vi "stop_gb_test_if_hp_test_fail.vi"(8 "error in (no error)":errorcluster, 9 "Message Queues in":T1, 11 "Pass/Fail":cluster{"PASS":bool, "FAIL":bool}) -> (0 "error out":errorcluster, 1 "Message Queues out":T1, 3 "Fail?":bool)   [LabVIEW 2015]
uses:
  support/Message Queue/All Message Queues.ctl
  support/Message Queue/Message Cluster.ctl
  support/Message Queue/Enqueue Message (Array).vi
  support/Message Queue/Message Queue.lvlib
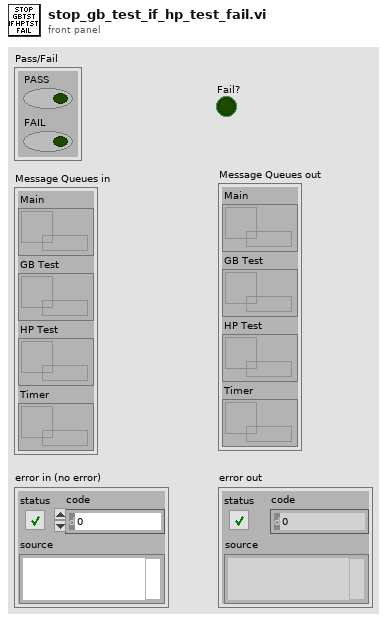
[diagram p1: front panel]
types:
  T1 = typedef "Message Queue.lvlib/All Message Queues.ctl" = cluster{"Main":refnum<queue>, "GB Test":refnum<queue>, "HP Test":refnum<queue>, "Timer":refnum<queue>}
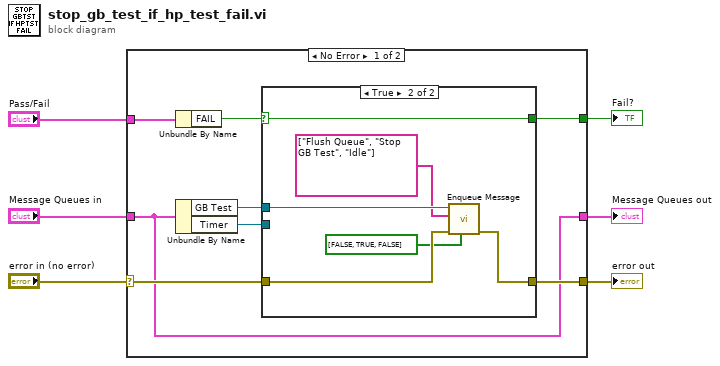
[diagram p0: block diagram]
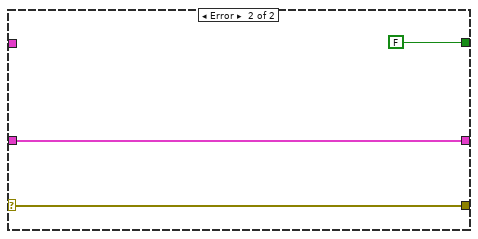
[diagram p3: hidden frame]
diagram:
  n1 = case shown="No Error" "error in (no error)" {
    selector: "error in (no error)" -> [w10 w25]
    tunnel: "Pass/Fail" -> [w13 _]
    tunnel: "Message Queues in" -> [w7 w23]
    tunnel: [w9 w25] -> w3
    tunnel: [w8 FALSE] -> w2
    tunnel: [w7 w23] -> w1
    frame No Error {
      n2 = Unbundle By Name(w13) -> ("FAIL"=w14:bool)
      n3 = Unbundle By Name(w7) -> ("GB Test"=w12:refnum<queue>, "Timer"=w11:refnum<queue>)
      n4 = case shown="True" w14 {
        selector: w14 -> [w16 w17]
        tunnel: w12 -> [_ w22]
        tunnel: w11 -> [_ _]
        tunnel: w10 -> [w15 w20]
        tunnel: [w15 w18] -> w9
        tunnel: [w16 w17] -> w8
        frame False {
        }
        frame True {
          n5 = call-poly "Enqueue Message.vi"("Priority Message? Array"=bool[] [FALSE, TRUE, FALSE], "error in (no error)"=w20, "Message Array"=string[] ["Flush Queue", "Stop GB Test", "Idle"], "Message Queue"=w22) -> ("error out"=w18:errorcluster)  [unwired: 6 in, 1 out]
        }
      }
    }
    frame Error {
    }
  }
  "error out" <- w3
  "Fail?" <- w2
  "Message Queues out" <- w1
